vi "_Read XIC.vi"(0 "file path":path, 1 "Offset":dbl, 2 "File Offset":dbl[](array[numeric]), 7 "Expt#":i32=1, 9 "MR#":i32=1, 11 "error in (no error)":errorcluster) -> (4 "Data":T6, 6 "Expt# Out":i32=1, 8 "MR# Out":i32=1, 10 "Version":i32, 15 "error out":errorcluster)   [LabVIEW 2015]
uses:
  Type/_Data.ctl
  Type/_XML Expt.ctl
  Type/_XML Lens.ctl
  Type/_Mass Range Property.ctl
  Type/_Mass Range Parameters.ctl
  Type/_RT Res Type.ctl
  Type/_GUI Method.ctl
  Type/_Lens Property.ctl
  Type/_Run Mode.ctl
panel:
  out "Steps":i32[][](array[numeric])
  in  "AcqMethod":T1[](array[typedef]) {"ScanType" format="%#.6g"; "Mass Range"."Res" items=["High/High", "Medium/Medium", "Low/Low", "High/Medium", "High/Low", "Medium/High", "Medium/Low", "Low/High", "Low/Medium"]}
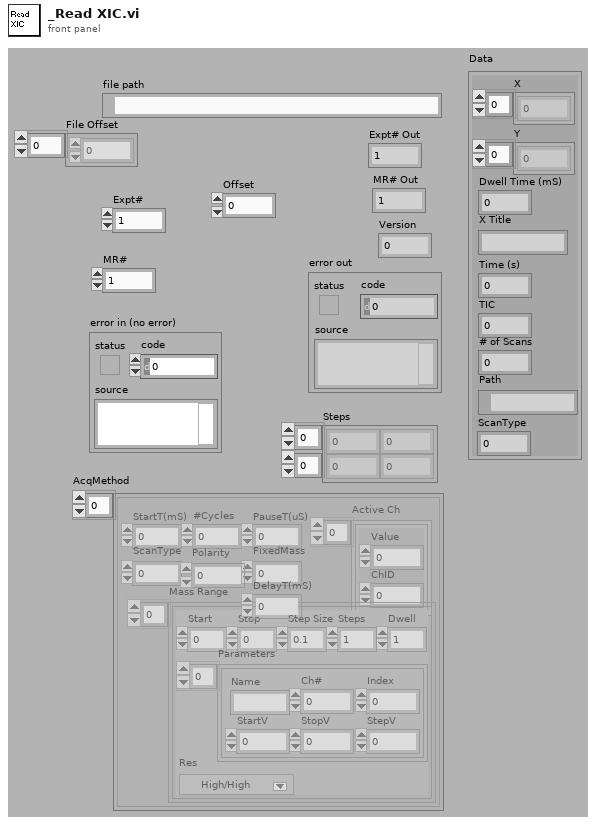
[diagram p1: front panel]
types:
  T1 = typedef "_XML Expt.ctl" = cluster{"StartT(mS)":i32, "#Cycles":i32, "PauseT(uS)":i32, "ScanType":i32, "Polarity":u8, "FixedMass":dbl, "DelayT(mS)":i32, "Active Ch":T2[], "Mass Range":T3[]}
  T2 = typedef "_XML Lens.ctl" = cluster{"Value":dbl, "ChID":u8}
  T3 = typedef "_Mass Range Property.ctl" = cluster{"Start":dbl, "Stop":dbl, "Step Size":dbl, "Steps":i32, "Dwell":dbl, "Parameters":T4[], "Res":T5}
  T4 = typedef "_Mass Range Parameters.ctl" = cluster{"Name":string, "Ch#":u8, "StartV":dbl, "StopV":dbl, "StepV":dbl, "Index":u8}
  T5 = typedef "_RT Res Type.ctl" = u16
  T6 = typedef "_Data.ctl" = cluster{"X":dbl[], "Y":dbl[], "Dwell Time (mS)":dbl, "X Title":string, "Time (s)":dbl, "TIC":u32, "# of Scans":i32, "Path":path, "ScanType":i32}
  T7 = typedef "_GUI Method.ctl" = cluster{"Lenses":T8[], "Mass Ranges":T3[], "Acquire":bool, "MCA":bool, "Q1DC EN":bool, "Q1 POL":bool, "Q3 POL":bool, "Q1 RF  EN":bool, "Averaging":bool, "Log Scale":bool, "CPS":bool, "Unit":bool, "Data Path":path, "Run Mode":T9, "Fixed Mass (amu)":dbl, "Q3DC EN":bool, "Q3 RF  EN":bool, "Negative":bool}
  T8 = typedef "_Lens Property.ctl" = cluster{"Scan Type":u8, "Scans":i32, "Time 1":dbl, "Time 2":dbl, "Value 1":dbl, "Value 2":dbl, "Step Size":dbl}
  T9 = typedef "_Run Mode.ctl" = enum16{"MRM (Q1/Q2)", "Q1 Scan", "Q1 SRM", "Q2 Scan", "Q2 SRM", "Product Scan", "Precursor Scan", "Neutral Loss", "Neutral Gain"}
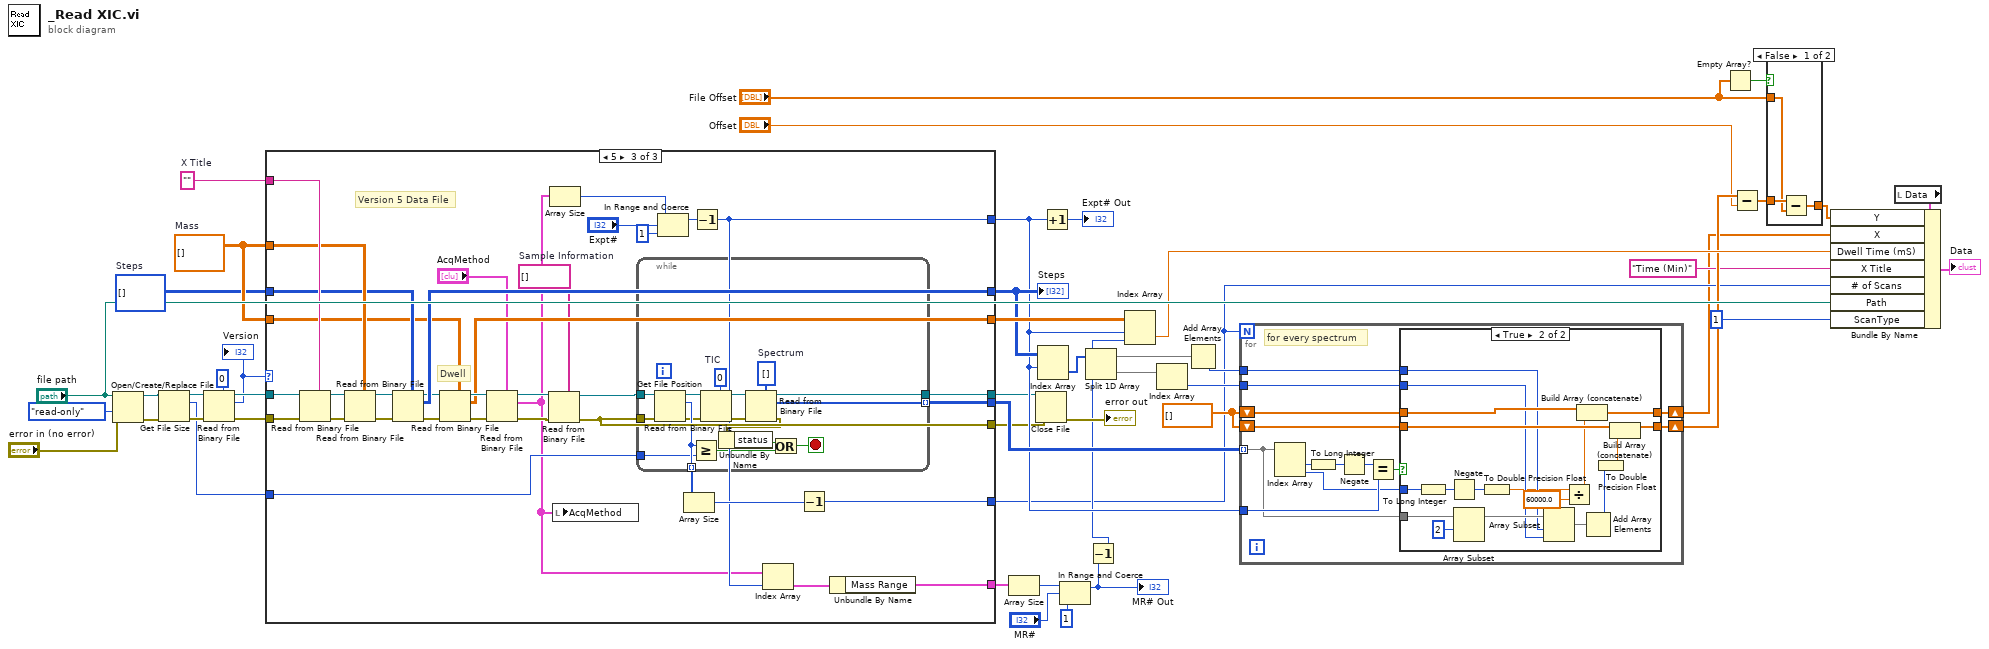
[diagram p0: block diagram]
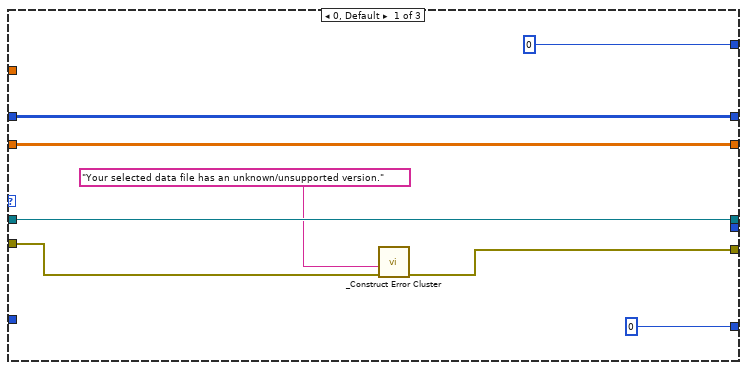
[diagram p4: hidden frame]
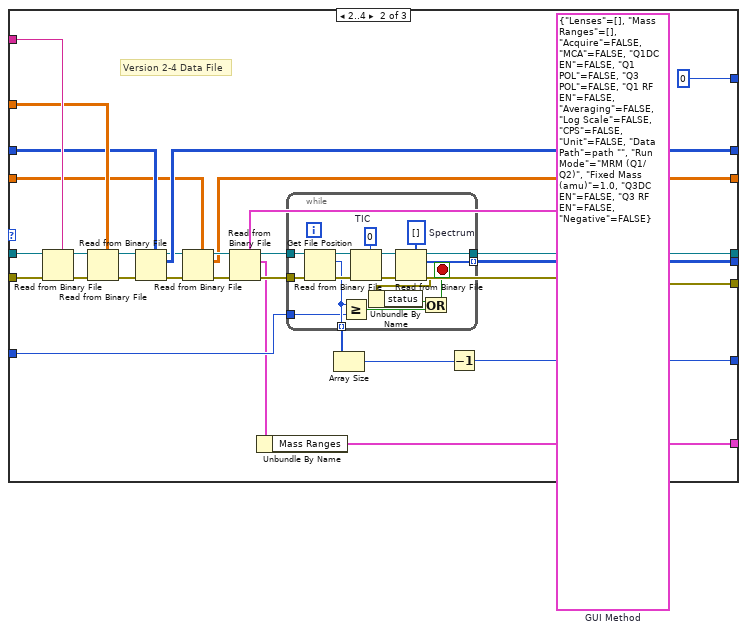
[diagram p5: hidden frame]
diagram:
  w16 = dbl[] [] ("subarray")
  w30 = ""  # X Title
  w31 = i32[][] []  # Steps
  w32 = dbl[][] []  # Mass
  n1 = Open/Create/Replace File(file path (use dialog)="file path", error in="error in (no error)", access (0:read/write)=enum16{"read/write", "read-only", "write-only"}."read-only") -> (refnum out=w43:refnum<file>, error out=w42:errorcluster)  [unwired: 4 out]
  n2 = Get File Size ("EOF")(file=w43, error in=w42) -> (refnum out=w39:refnum<file>, size (in bytes)=w35:i64, 0:w38:errorcluster)
  n3 = Read from Binary File(5:0 ("pos offset (0)"), 8:w38, 11:w39) -> (0:w36:errorcluster, 2:w29:i32, 3:w37:refnum<file>)  [unwired: 4 out]
  "Version" <- w29
  n4 = case shown="5" w29 {
    tunnel: w36 -> [w55 w82 w134]
    tunnel: w37 -> [w56 w81 w133]
    tunnel: [0 w63 w117] -> w7
    tunnel: [w56 w67 w120] -> w13
    tunnel: [w53 w66 w113] -> w12
    tunnel: w35 -> [_ w62 w116]
    tunnel: [w50 w78 w130] -> w23
    tunnel: w30 -> [_ w77 w129]
    tunnel: w32 -> [_ w76 w128]
    tunnel: w31 -> [w50 w75 w127]
    tunnel: w32 -> [w51 w69 w122]
    tunnel: [w51 w68 w121] -> w34
    tunnel: [0 ("lower limit") 0 ("lower limit") w105] -> w17
    tunnel: [_ w58 w102] -> w27
    tunnel: [_ w57 w101] -> w18
    frame 0, Default {
      n5 = call "_Construct Error Cluster.vi"("error in"=w55, "reason"="Your selected data file has an unknown/unsupported version.") -> ("error out"=w53:errorcluster)  [unwired: 2 in, 3 out]
    }
    frame 2..4 {
      w61 = T7 {"Lenses"=[], "Mass Ranges"=[], "Acquire"=FALSE, "MCA"=FALSE, "Q1DC EN"=FALSE, "Q1 POL"=FALSE, "Q3 POL"=FALSE, "Q1 RF  EN"=FALSE, "Averaging"=FALSE, "Log Scale"=FALSE, "CPS"=FALSE, "Unit"=FALSE, "Data Path"=path "", "Run Mode"=enum."MRM (Q1/Q2)", "Fixed Mass (amu)"=1.0, "Q3DC EN"=FALSE, "Q3 RF  EN"=FALSE, "Negative"=FALSE}  # GUI Method
      # "Version 2-4 Data File"
      n6 = Read from Binary File(5:w77, 8:w82, 11:w81) -> (0:w84:errorcluster, 3:w80:refnum<file>)  [unwired: 5 out]
      n7 = Read from Binary File(5:w76, 8:w84, 11:w80) -> (0:w83:errorcluster, 3:w79:refnum<file>)  [unwired: 5 out]
      n8 = Read from Binary File(5:w75, 8:w83, 11:w79) -> (0:w71:errorcluster, 2:w78:i32[][], 3:w72:refnum<file>)  [unwired: 4 out]
      n9 = Read from Binary File(5:w69, 8:w71, 11:w72) -> (0:w73:errorcluster, 2:w68:dbl[][], 3:w70:refnum<file>)  [unwired: 4 out]
      n10 = Read from Binary File(5:w61, 8:w73, 11:w70) -> (0:w66:errorcluster, 2:w59:T7, 3:w74:refnum<file>)  [unwired: 4 out]
      n11 = Unbundle By Name(w59) -> ("Mass Ranges"=w58:T3[])
      n12 = while {
        tunnel: w74 -> [w100]
        tunnel: w66 -> [w99]
        tunnel: [w97] -> w67
        tunnel: [w96] -> w65 mode=indexing
        tunnel: w62 -> [w95]
        tunnel: [w85] -> w57 mode=indexing
        stop <- w92 stop-if-true
        w87 = u32 0  # TIC
        w98 = u32[] []  # Spectrum
        n13 = Get File Position(4:w99, 7:w100) -> (0:w88:errorcluster, 2:w96:i64, 3:w90:refnum<file>)
        n14 = Greater Or Equal?(x=w96, y=w95) -> (x >= y?=w93:bool)
        n15 = Read from Binary File(5:w87, 8:w88, 11:w90) -> (0:w91:errorcluster, 3:w89:refnum<file>)  [unwired: 5 out]
        n16 = Read from Binary File(5:w98, 8:w91, 11:w89) -> (0:w86:errorcluster, 2:w85:u32[], 3:w97:refnum<file>)  [unwired: 4 out]
        n17 = Unbundle By Name(w86) -> ("status"=w94:bool)
        n18 = Or(x=w94, y=w93) -> (x .or. y?=w92:bool)
      }
      n19 = Array Size(array=w65) -> (size(s)=w64:i32)
      n20 = Decrement(x=w64) -> (x-1=w63:i32)
    }
    frame 5 {
      w111 = string[] []  # Sample Information
      # "Dwell"
      # "Version 5 Data File"
      n21 = Read from Binary File(5:w129, 8:w134, 11:w133) -> (0:w136:errorcluster, 3:w132:refnum<file>)  [unwired: 5 out]
      n22 = Read from Binary File(5:w128, 8:w136, 11:w132) -> (0:w135:errorcluster, 3:w131:refnum<file>)  [unwired: 5 out]
      n23 = Read from Binary File(5:w127, 8:w135, 11:w131) -> (0:w124:errorcluster, 2:w130:i32[][], 3:w125:refnum<file>)  [unwired: 4 out]
      n24 = Read from Binary File(5:w122, 8:w124, 11:w125) -> (0:w126:errorcluster, 2:w121:dbl[][], 3:w123:refnum<file>)  [unwired: 4 out]
      n25 = Read from Binary File(5:"AcqMethod", 8:w126, 11:w123) -> (0:w112:errorcluster, 2:w103:T1[], 3:w115:refnum<file>)  [unwired: 4 out]
      n26 = Read from Binary File(5:w111, 8:w112, 11:w115) -> (0:w113:errorcluster, 3:w114:refnum<file>)  [unwired: 5 out]
      n27 = Array Size(array=w103) -> (size(s)=w106:i32)
      n28 = local write "AcqMethod"(w103) -> ()
      n29 = while {
        tunnel: w114 -> [w152]
        tunnel: w113 -> [w151]
        tunnel: [w149] -> w120
        tunnel: [w148] -> w119 mode=indexing
        tunnel: w116 -> [w147]
        tunnel: [w137] -> w101 mode=indexing
        stop <- w144 stop-if-true
        w139 = u32 0  # TIC
        w150 = u32[] []  # Spectrum
        n30 = Get File Position(4:w151, 7:w152) -> (0:w140:errorcluster, 2:w148:i64, 3:w142:refnum<file>)
        n31 = Greater Or Equal?(x=w148, y=w147) -> (x >= y?=w145:bool)
        n32 = Read from Binary File(5:w139, 8:w140, 11:w142) -> (0:w143:errorcluster, 3:w141:refnum<file>)  [unwired: 5 out]
        n33 = Read from Binary File(5:w150, 8:w143, 11:w141) -> (0:w138:errorcluster, 2:w137:u32[], 3:w149:refnum<file>)  [unwired: 4 out]
        n34 = Unbundle By Name(w138) -> ("status"=w146:bool)
        n35 = Or(x=w146, y=w145) -> (x .or. y?=w144:bool)
      }
      n36 = In Range and Coerce(upper limit=w106, x="Expt#", lower limit=1) -> (coerced(x)=w107:i32)  [unwired: 1 out]
      n37 = Array Size(array=w119) -> (size(s)=w118:i32)
      n38 = Decrement(x=w107) -> (x-1=w105:i32)
      n39 = Index Array(array=w103, index=w105) -> (element=w104:T1)
      n40 = Decrement(x=w118) -> (x-1=w117:i32)
      n41 = Unbundle By Name(w104) -> ("Mass Range"=w102:T3[])
    }
  }
  "Steps" <- w23
  n42 = Array Size(array=w27) -> (size(s)=w25:i32)
  n43 = Close File(refnum=w13, error in=w12) -> (error out=→"error out":errorcluster)  [unwired: 1 out]
  n44 = Index Array(array=w23, index (row)=w17) -> (element=w22:i32[])  [unwired: 1 in]
  n45 = Increment(x=w17) -> (x+1=→"Expt# Out":i32)
  n46 = In Range and Coerce(upper limit=w25, x="MR#", lower limit=1) -> (coerced(x)=w21:i32)  [unwired: 1 out]
  "MR# Out" <- w21
  n47 = Decrement(x=w21) -> (x-1=w11:i32)
  n48 = Split 1D Array(array=w22, index=w11) -> (first subarray=w20:i32[], second subarray=w19:i32[])
  n49 = Index Array(array=w34, index (row)=w17, index (col)=w11) -> (element=w33:dbl)
  n50 = Index Array(array=w19) -> (element=w14:i32)  [unwired: 1 in]
  n51 = Add Array Elements(numeric array=w20) -> (sum=w15:i32)
  n52 = for {
    N: w7 -> [_]
    tunnel: w18 -> [w155] mode=indexing
    shift-right: [w158] -> w4
    shift-left: w16 -> [w160]
    shift-right: [w157] -> w10
    shift-left: w16 -> [w159]
    tunnel: w17 -> [w162]
    tunnel: w15 -> [w154]
    tunnel: w14 -> [w153]
    # "for every spectrum"
    n53 = Index Array(array=w155) -> (element #1=w164:u32, element #2=w156:u32)  [unwired: 2 in]
    n54 = To Long Integer(number=w164) -> (32bit integer=w165:i32)
    n55 = Negate(x=w165) -> (-x=w163:i32)
    n56 = Equal?(x=w163, y=w162) -> (x = y?=w161:bool)
    n57 = case shown="True" w161 {
      tunnel: w160 -> [w167 w183]
      tunnel: w159 -> [w166 w176]
      tunnel: [w167 w181] -> w158
      tunnel: [w166 w175] -> w157
      tunnel: w156 -> [_ w184]
      tunnel: w155 -> [_ w179]
      tunnel: w154 -> [_ w172]
      tunnel: w153 -> [_ w171]
      frame False {
      }
      frame True {
        n58 = To Long Integer(number=w184) -> (32bit integer=w185:i32)
        n59 = Negate(x=w185) -> (-x=w182:i32)
        n60 = Array Subset(array=w179, index=2) -> (w178:u32[])  [unwired: 1 in]
        n61 = To Double Precision Float(number=w182) -> (double precision float=w169:dbl)
        n62 = Array Subset(array=w178, index=w172, length=w171) -> (w177:u32[])
        n63 = Divide(x=w169, y=60000.0) -> (x/y=w168:dbl)
        n64 = Build Array (concatenate)(w183, w168) -> (w181:dbl[])
        n65 = Add Array Elements(numeric array=w177) -> (sum=w173:u32)
        n66 = To Double Precision Float(number=w173) -> (double precision float=w174:dbl)
        n67 = Build Array (concatenate)(w176, w174) -> (w175:dbl[])
      }
    }
  }
  n68 = Empty Array?(array="File Offset") -> (empty?=w2:bool)
  n69 = Subtract(x=w10, y="Offset") -> (x-y=w5:dbl[])
  n70 = case shown="False" w2 {
    tunnel: w5 -> [w188 w189]
    tunnel: "File Offset" -> [w187 _]
    tunnel: [w186 w189] -> w1
    frame False {
      n71 = Subtract(x=w188, y=w187) -> (x-y=w186:dbl[])
    }
    frame True {
    }
  }
  n72 = local read "Data"() -> (w46:T6)
  n73 = Bundle By Name(cluster=w46, "Y"=w1, "X"=w4, "Dwell Time (mS)"=w33, "X Title"="Time (Min)", "# of Scans"=w7, "Path"="file path", "ScanType"=1) -> (→"Data":T6)
